vi "Generate multi tone waveform.vi"(6 "hardware commands sync queue":T2, 8 "error in":errorcluster, 9 "measurement configuration":T1={"Full scale range"=2.825, "Channel name"="", "Analog source resource name"="", "IMD standard"=enum."CCIF (11 kHz, 12 kHz, 1:1)", "Low frequency"=14000.0, "High frequency"=15000.0, "Amplitude ratio"=1.0, "Amplitude"=-1.0, "Protocol capture resource name"="", "Data line"=0, "Channel"=0, "Sample rate"=44100.0, "Measurement duration"=0.1, "Frame sync edge for Channel 0"=enum."Falling", "Channel count per frame"=2, "Channel length"=32, "Bit depth"=24, "Channel 0 offset"=1, "Endianness"=enum."MSB First", "Data Justification"=enum."Left Justified", "Frame length"=64, "Frame sync pulse width"=32, "Bit clock edge  sync"=enum."Falling"} {"High frequency" format="%#_pHz"; "Low frequency" format="%#_pHz"}, 10 "Sample Rate (Hz)":dbl=51200.0, 11 "task/channels in":refnum<k21>) -> (0 "error out":errorcluster, 3 "task out":refnum<k21>)   [LabVIEW 2021, in "IMD_Audio ADC.lvlib"]
uses:
  IMD_Audio ADC.lvlib
  shared/controls/Sync Commands Queue Ref.ctl
  shared/controls/Sync Commands.ctl
  Measurement Configuration.ctl
  <vilib>/addons/_NISVFA/_Generation/Signal Generation/SV Signal/sv_System Timing Model.ctl
  <vilib>/DAQmx/write.llb/DAQmx Write (Analog 1D Wfm NChan NSamp).vi
  <vilib>/addons/_NISVFA/_Generation/Signal Generation/SV Multitone/SV Multitone.lvclass
  C:/Program Files/National Instruments/LabVIEW 2021/vi.lib/addons/_NISVFA/_Generation/Signal Generation/SV Signal/SV Signal.lvclass
  <vilib>/addons/_NISVFA/_Generation/Signal Generation/SV Multitone/Configure Multitone (Custom).vi
  <vilib>/addons/_NISVFA/_Generation/Signal Generation/SV Signal/Write Sample Rate.vi
  <vilib>/addons/_NISVFA/_Generation/Signal Generation/SV Signal/Write System Timing Model.vi
  <vilib>/addons/_NISVFA/_Generation/Signal Generation/SV Signal/Write Ramp Parameters.vi
  <vilib>/DAQmx/miscellaneous.llb/DAQmx Fill In Error Info.vi
  <vilib>/addons/_NISVFA/_Generation/Signal Generation/SV Signal/SV Signal.lvclass
  shared/controls/Audio ADC Controls.lvlib
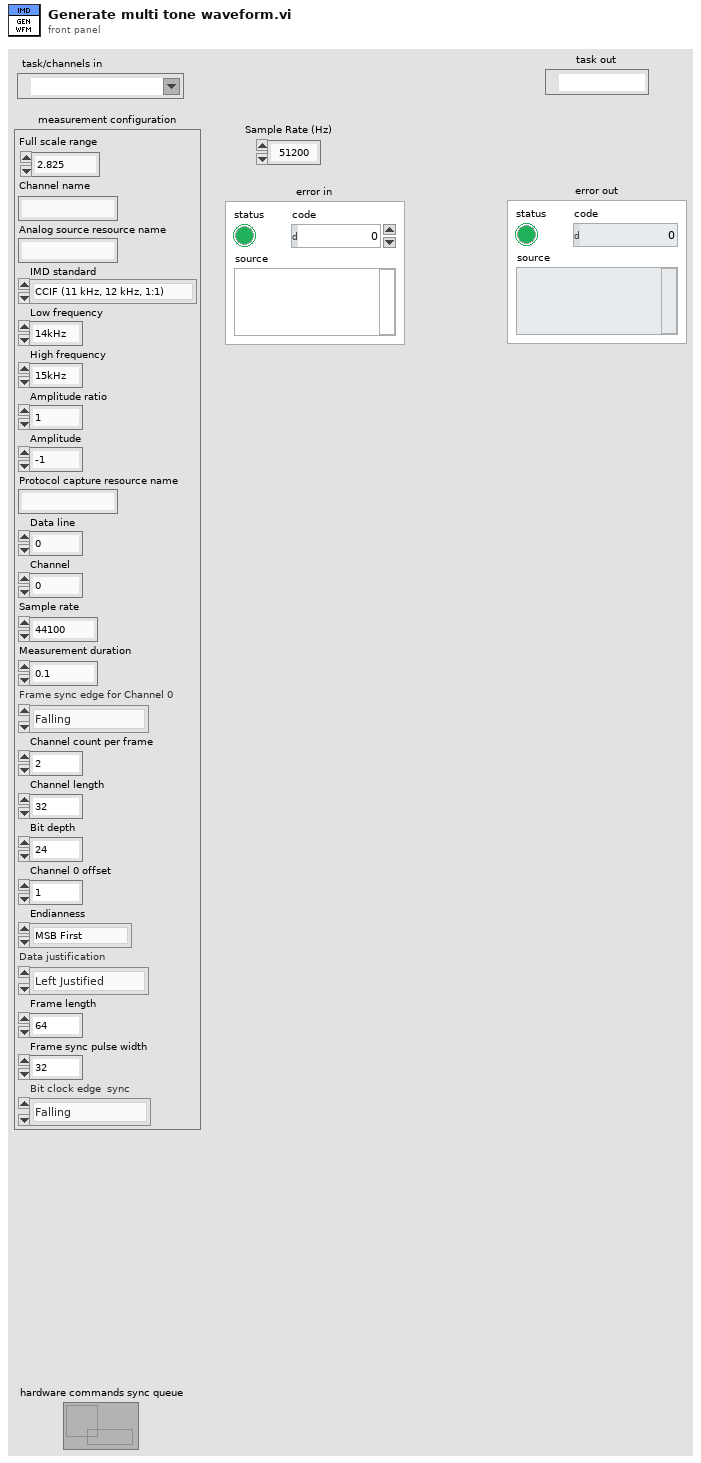
[diagram p1: front panel]
types:
  T1 = typedef "IMD_Audio ADC.lvlib/Measurement Configuration.ctl" = cluster{"Full scale range":dbl, "Channel name":string, "Analog source resource name":string, "IMD standard":enum32{"SMPTE (60 Hz, 7000 Hz, 4:1)", "DIN (250 Hz, 8000 Hz, 4:1)", "CCIF (11 kHz, 12 kHz, 1:1)", "CCIF (19 kHz, 20 kHz, 1:1)", "Custom"}, "Low frequency":dbl, "High frequency":dbl, "Amplitude ratio":dbl, "Amplitude":dbl, "Protocol capture resource name":string, "Data line":u32, "Channel":u32, "Sample rate":dbl, "Measurement duration":dbl, "Frame sync edge for Channel 0":enum32{"Rising", "Falling"}, "Channel count per frame":u32, "Channel length":u32, "Bit depth":u32, "Channel 0 offset":u32, "Endianness":enum32{"MSB First", "LSB First"}, "Data Justification":enum32{"Left Justified", "Right Justified"}, "Frame length":u32, "Frame sync pulse width":u32, "Bit clock edge  sync":enum32{"Rising", "Falling"}}
  T2 = typedef "Audio ADC Controls.lvlib/Sync Commands Queue Ref.ctl" = refnum<queue>
  T3 = cluster{"profile":enum16{"Linear", "Half cosine"}, "durations [s]":cluster{"ramp-up":dbl, "transition":dbl, "ramp-down":dbl}}
  T4 = typedef "audio adc controls.lvlib/Sync Commands.ctl" = enum16{"NoAction", "GenerationStarted", "AcquisitionCompleted", "GenerationErrored"}
  T5 = typedef "SV Signal.lvclass/sv_System Timing Model.ctl" = i64
  T6 = enum32{"SMPTE (60 Hz, 7000 Hz, 4:1)", "DIN (250 Hz, 8000 Hz, 4:1)", "CCIF (11 kHz, 12 kHz, 1:1)", "CCIF (19 kHz, 20 kHz, 1:1)", "Custom"}
  T7 = typedef "Audio ADC Controls.lvlib/Sync Commands.ctl" = enum16{"NoAction", "GenerationStarted", "AcquisitionCompleted", "GenerationErrored"}
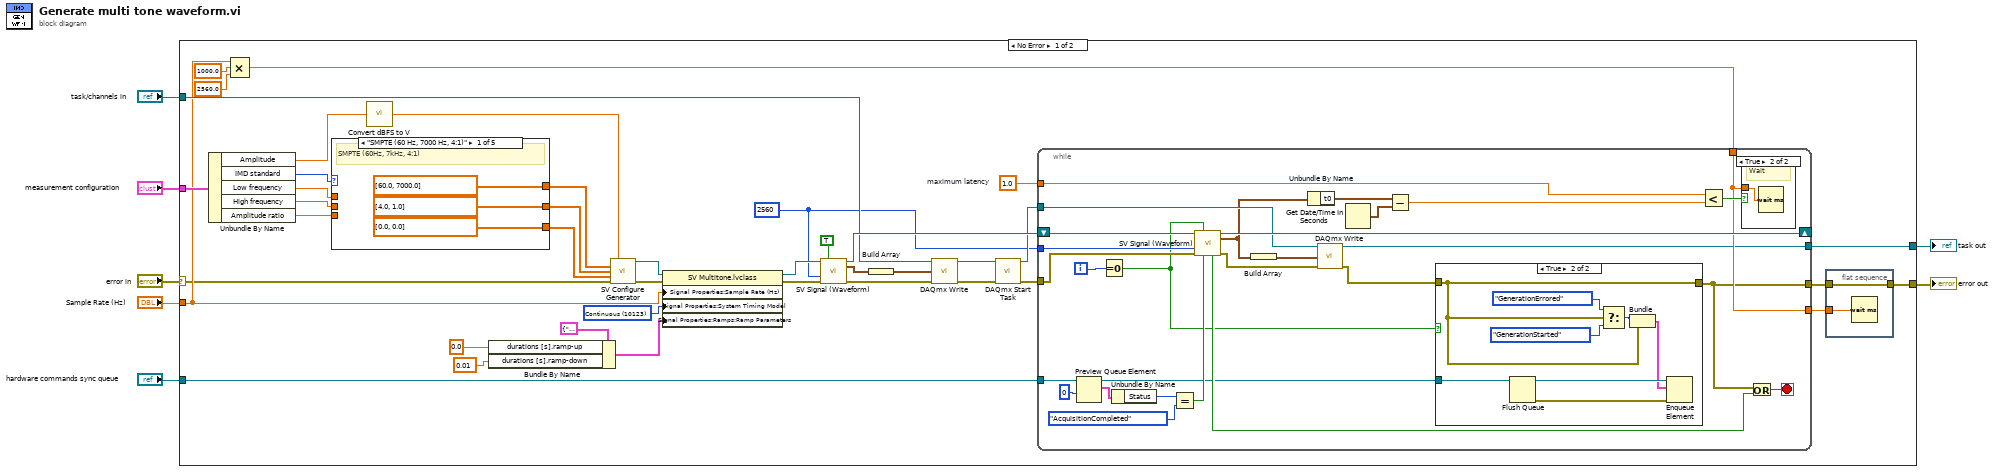
[diagram p0: block diagram]
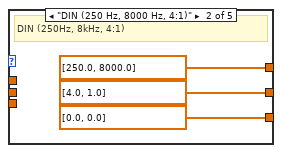
[diagram p4: hidden frame]
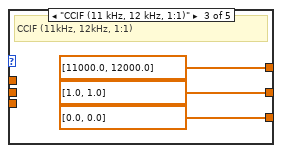
[diagram p5: hidden frame]
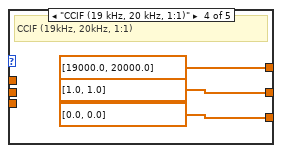
[diagram p6: hidden frame]
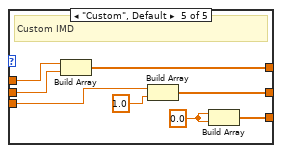
[diagram p7: hidden frame]
diagram:
  n1 = case shown="No Error" "error in" {
    selector: "error in" -> [w8 w110]
    tunnel: [w11 w110] -> w6
    tunnel: "measurement configuration" -> [w48 _]
    tunnel: "task/channels in" -> [w25 w109]
    tunnel: "Sample Rate (Hz)" -> [w16 _]
    tunnel: [w10 w109] -> w3
    tunnel: "hardware commands sync queue" -> [w9 _]
    frame No Error {
      w18 = 1.0  # maximum latency
      w34 = T5 10123 items=["Finite"=10178, "-"=-1, "Continuous"=10123, "-"=-2, "Settled"=110123, "Averaged"=210123, "Discrete Sweep"=310123, "Continuous Sweep"=410123] ("System Timing Model")
      w19 = 2560 ("samples")
      n2 = Unbundle By Name(w48) -> ("Amplitude"=w43:dbl, "IMD standard"=w47:T6, "Low frequency"=w46:dbl, "High frequency"=w45:dbl, "Amplitude ratio"=w44:dbl)
      n3 = Compound Arithmetic op=MULTIPLY(w16, 1000.0 ("value"), 2560.0 ("value")) -> (w17:dbl)
      n4 = case shown="\"SMPTE (60 Hz, 7000 Hz, 4:1)\"" w47 {
        tunnel: [dbl[] [60.0, 7000.0] ("source settings.frequencies") dbl[] [250.0, 8000.0] ("source settings.frequencies") dbl[] [11000.0, 12000.0] ("source settings.frequencies") dbl[] [19000.0, 20000.0] ("source settings.frequencies") w106] -> w42
        tunnel: [dbl[] [4.0, 1.0] ("source settings.frequencies") dbl[] [4.0, 1.0] ("source settings.frequencies") dbl[] [1.0, 1.0] ("source settings.frequencies") dbl[] [1.0, 1.0] ("source settings.frequencies") w105] -> w41
        tunnel: [dbl[] [0.0, 0.0] ("source settings.frequencies") dbl[] [0.0, 0.0] ("source settings.frequencies") dbl[] [0.0, 0.0] ("source settings.frequencies") dbl[] [0.0, 0.0] ("source settings.frequencies") w104] -> w40
        tunnel: w46 -> [_ _ _ _ w103]
        tunnel: w45 -> [_ _ _ _ w102]
        tunnel: w44 -> [_ _ _ _ w101]
        frame "SMPTE (60 Hz, 7000 Hz, 4:1)" {
          # "SMPTE (60Hz, 7kHz, 4:1)"
        }
        frame "DIN (250 Hz, 8000 Hz, 4:1)" {
          # "DIN (250Hz, 8kHz, 4:1)"
        }
        frame "CCIF (11 kHz, 12 kHz, 1:1)" {
          # "CCIF (11kHz, 12kHz, 1:1)"
        }
        frame "CCIF (19 kHz, 20 kHz, 1:1)" {
          # "CCIF (19kHz, 20kHz, 1:1)"
        }
        frame "Custom", Default {
          w107 = 0.0 ("element")
          # "Custom IMD"
          n5 = Build Array(w103, w102) -> (w106:dbl[])
          n6 = Build Array(w101, 1.0 ("element")) -> (w105:dbl[])
          n7 = Build Array(w107, w107) -> (w104:dbl[])
        }
      }
      n8 = call "Convert dBFS to V.vi"("Amplitude (dBFS)"=w43) -> ("Amplitude (V)"=w39:dbl)
      n9 = Bundle By Name(cluster=T3 {"profile"=enum."Linear", "durations [s]"={"ramp-up"=0.0, "transition"=0.0, "ramp-down"=0.0}} ("Ramp Parameters:All Elements"), "durations [s].ramp-up"=0.0, "durations [s].ramp-down"=0.01) -> (w32:T3)
      n10 = call-poly <vilib>:"SV Configure Generator.vi"("overall amplitude"=w39, "frequencies [Hz]"=w42, "amplitudes"=w41, "phases [deg]"=w40, "error in (no error)"=w8) -> ("signal configuration"=w38:refnum<class "SV Multitone.lvclass">, "error out"=w36:errorcluster)  [unwired: 8 in, 1 out]
      n11 = property class="SV Multitone.lvclass"(reference=w38, error in=w36, "Signal Properties:Sample Rate (Hz)"=w16, "Signal Properties:System Timing Model"=w34, "Signal Properties:Ramps:Ramp Parameters"=w32) -> (reference out=w37:refnum<class "SV Multitone.lvclass">, error out=w35:errorcluster)
      n12 = call-dynamic "SV Signal (Waveform).vi"("signal configuration"=w37, "reset"=TRUE, "samples"=w19, "error in (no error)"=w35) -> ("signal configuration"=w28:refnum<class "SV Multitone.lvclass">, "output waveform"=w29:waveform(dbl), "error out"=w21:errorcluster)  [unwired: 6 in, 3 out]
      n13 = Build Array(w29) -> (w27:waveform(dbl)[])
      n14 = call-poly <vilib>:"DAQmx Write.vi"("task/channels in"=w25, "data"=w27, "error in"=w21) -> ("task out"=w26:refnum<k21>, "error out"=w22:errorcluster)  [unwired: 10 in, 1 out]
      n15 = call <vilib>:"DAQmx Start Task.vi"("task/channels in"=w26, "error in"=w22) -> ("task out"=w23:refnum<k21>, "error out"=w20:errorcluster)  [unwired: 12 in]
      n16 = while {
        shift-right: [w77] -> _
        shift-left: w28 -> [w78]
        tunnel: w19 -> [w68]
        tunnel: w23 -> [w74]
        tunnel: [w54] -> w10
        tunnel: [w53] -> w12
        tunnel: w18 -> [w70]
        tunnel: w17 -> [w65]
        tunnel: [w65] -> w13
        tunnel: w20 -> [w64]
        tunnel: w9 -> [w56]
        i -> [w60]
        stop <- w76 stop-if-true
        n17 = Preview Queue Element(queue=w56, timeout in ms (-1)=0) -> (queue out=w51:T2, element=w61:cluster{"Status":T7, "Error":errorcluster})  [unwired: 1 in, 2 out]
        n18 = Equal To 0?(x=w60) -> (x = 0?=w52:bool)
        n19 = Unbundle By Name(w61) -> ("Status"=w59:T7)
        n20 = Equal?(x=w59, y=Sync_Commands."AcquisitionCompleted") -> (x = y?=w57:bool)
        n21 = call-dynamic "SV Signal (Waveform).vi"("signal configuration"=w78, "reset"=w52, "samples"=w68, "error in (no error)"=w64, "stop"=w57) -> ("signal configuration"=w77:refnum<class "SV Multitone.lvclass">, "output waveform"=w67:waveform(dbl), "done"=w75:bool, "error out"=w63:errorcluster)  [unwired: 5 in, 2 out]
        n22 = Build Array(w67) -> (w66:waveform(dbl)[])
        n23 = Unbundle By Name(w67) -> ("t0"=w73:timestamp)
        n24 = call-poly <vilib>:"DAQmx Write.vi"("task/channels in"=w74, "data"=w66, "error in"=w63) -> ("task out"=w54:refnum<k21>, "error out"=w55:errorcluster)  [unwired: 10 in, 1 out]
        n25 = Get Date/Time In Seconds() -> (seconds since 1Jan1904=w72:timestamp)
        n26 = Subtract(x=w73, y=w72) -> (x-y=w71:dbl)
        n27 = case shown="True" w52 {
          tunnel: w51 -> [_ w87]
          tunnel: w55 -> [w79 w81]
          tunnel: [w79 w81] -> w53
          frame False {
          }
          frame True {
            n28 = Flush Queue(queue=w87) -> (queue out=w86:T2, error out=w85:errorcluster)  [unwired: 1 in, 1 out]
            n29 = Select(t=Sync_Commands."GenerationErrored" ("element"), s=w81, f=Sync_Commands."GenerationStarted" ("element")) -> (s? t:f=w82:T4)
            n30 = Bundle("element"=w82, "error out"=w81) -> (w80:cluster{"element":T4, "error out":errorcluster})  [unwired: 1 in]
            n31 = Enqueue Element(queue=w86, element=w80, error in (no error)=w85) -> ()  [unwired: 1 in, 3 out]
          }
        }
        n32 = Less?(x=w70, y=w71) -> (x < y?=w69:bool)
        n33 = case shown="True" w69 {
          tunnel: w65 -> [_ w88]
          frame False {
          }
          frame True {
            # "Wait"
            n34 = Wait (ms)(milliseconds to wait=w88) -> ()  [unwired: 1 out]
          }
        }
        n35 = Or(x=w53, y=w75) -> (x .or. y?=w76:bool)
      }
      n36 = flat-sequence {
        tunnel: w13 -> [w50]
        tunnel: w12 -> [w49]
        tunnel: [w49] -> w11
        frame #0 {
          n37 = Wait (ms)(milliseconds to wait=w50) -> ()  [unwired: 1 out]
        }
      }
    }
    frame Error {
    }
  }
  "error out" <- w6
  "task out" <- w3
